vi "创建README.vi"(8 "错误输入":errorcluster, 10 "描述":string, 11 "基路径":path) -> (0 "错误输出":errorcluster, 3 "基路径":path)   [LabVIEW 2018]
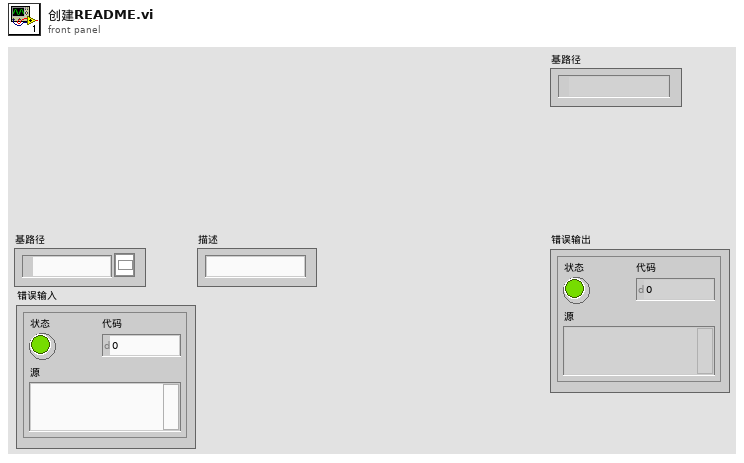
[diagram p1: front panel]
types:
  T1 = enum16{"open", "replace", "create", "open or create", "replace or create", "replace or create with confirmation"}
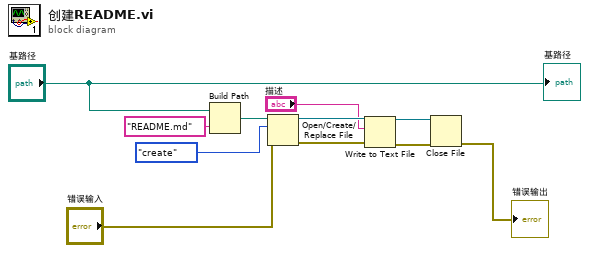
[diagram p0: block diagram]
diagram:
  n1 = Build Path(base path="基路径", name or relative path="README.md" ("名称或相对路径")) -> (appended path=w10:path)
  n2 = Open/Create/Replace File(file path (use dialog)=w10, error in="错误输入", operation (0:open)=T1."create" ("操作(0:open)")) -> (refnum out=w5:refnum<file>, error out=w8:errorcluster)  [unwired: 3 in, 1 out]
  n3 = Write to Text File(file (use dialog)=w5, text="描述", error in=w8) -> (refnum out=w3:refnum<file>, error out=w2:errorcluster)  [unwired: 1 in, 1 out]
  n4 = Close File(refnum=w3, error in=w2) -> (error out=→"错误输出":errorcluster)  [unwired: 1 out]
  "基路径" <- "基路径"
